vi "MPU_Stick_Plotter_Core_Test.vi"() -> ()   [LabVIEW 2017]
uses:
  <vilib>/Utility/miscctls.llb/LVPointDoubleTypeDef.ctl
  <vilib>/Utility/miscctls.llb/LVOffsetAndMultiplierTypeDef.ctl
  Controls/MPU_Stick_Plotter_Core_Commands.ctl
panel:
  out "Plot":cluster{"Values":dbl[], "Time (ms)":dbl[]}[](graph)
  in  "Channel Name":string="Channel A"
  in  "Offset & Range":T1
  out "Sample value":dbl
  out "Cursor.Cursor Position":T2
  in  "stop":bool
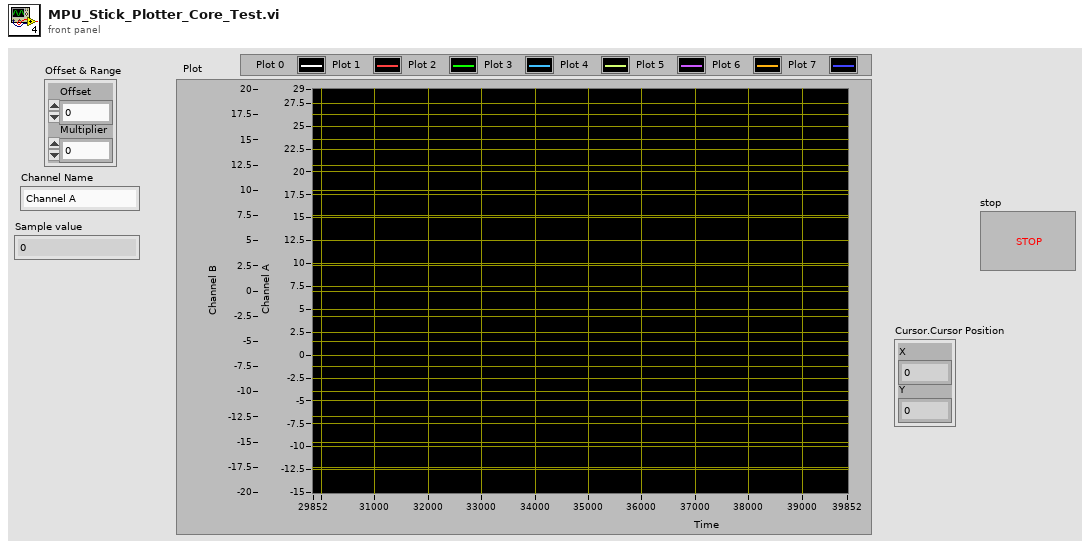
[diagram p1: front panel]
types:
  T1 = typedef "LVOffsetAndMultiplierTypeDef.ctl" = cluster{"Offset":dbl, "Multiplier":dbl}
  T2 = typedef "LVPointDoubleTypeDef.ctl" = cluster{"X":dbl, "Y":dbl}
  T3 = typedef "MPU_Stick_Plotter_Core_Commands.ctl" = enum16{"Initialize", "Add Channel", "Remove Channel", "Set Channel Minimum Value", "Set Channel Maximum Value", "Set Offset & Multiplier", "Get Offset & Multiplier", "Update Channel", "Get Cursor Data", "Clear", "Reset"}
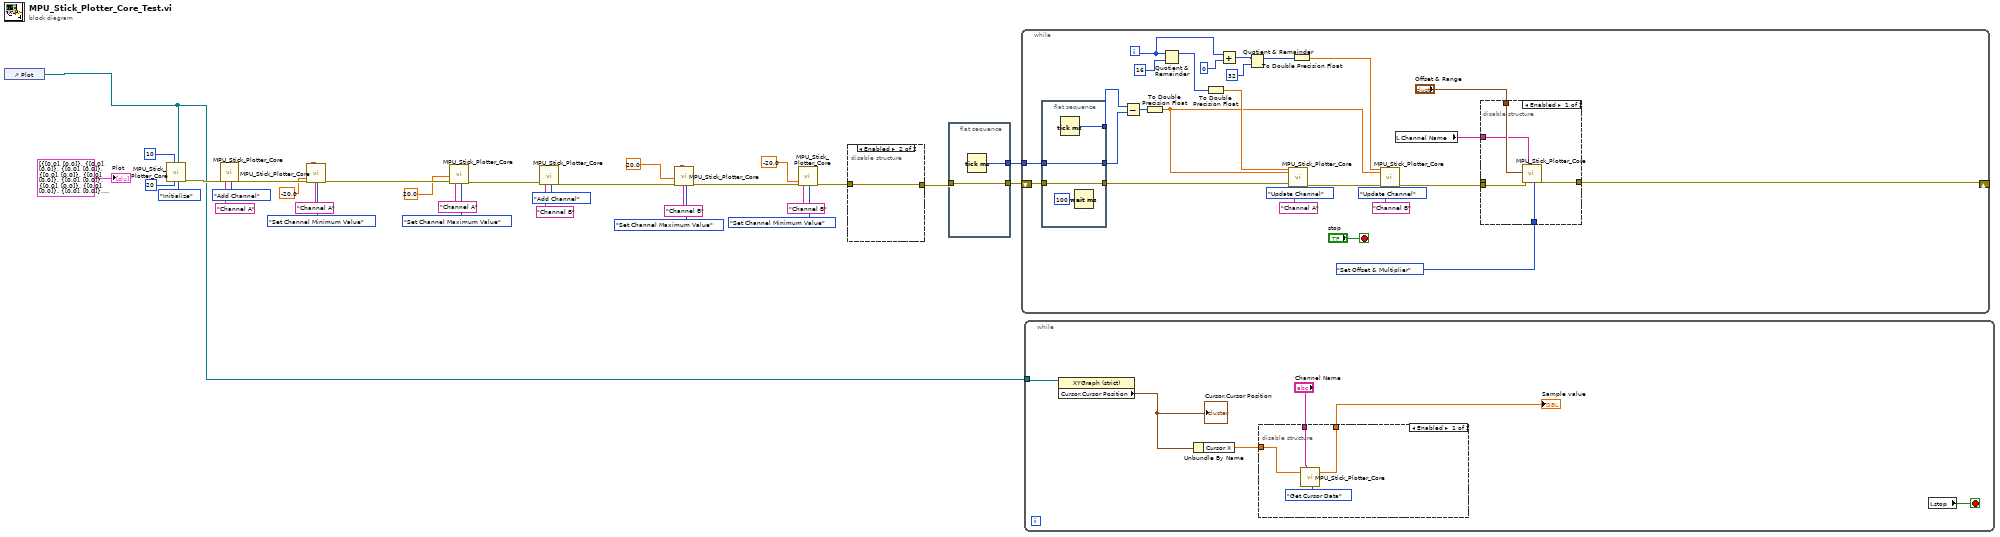
[diagram p0: block diagram]
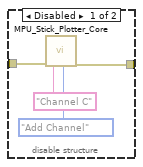
[diagram p2: hidden frame]
diagram:
  n1 = control-ref of="Plot"() -> (w1:refnum<vi>)
  n2 = call "MPU_Stick_Plotter_Core.vi"("Number of vertical divisions"=u16 10, "Number of horizontal divisions"=u16 20, "Plot reference"=w1, "Command"=MPU_Stick_Plotter_Core_Commands."Initialize") -> ("error out"=w30:errorcluster)  [unwired: 12 in, 3 out]
  n3 = call "MPU_Stick_Plotter_Core.vi"("error in (no error)"=w30, "Channel Name"="Channel A", "Command"=MPU_Stick_Plotter_Core_Commands."Add Channel") -> ("error out"=w25:errorcluster)  [unwired: 13 in, 3 out]
  n4 = call "MPU_Stick_Plotter_Core.vi"("Minimum"=-20.0, "error in (no error)"=w25, "Channel Name"="Channel A", "Command"=MPU_Stick_Plotter_Core_Commands."Set Channel Minimum Value") -> ("error out"=w21:errorcluster)  [unwired: 12 in, 3 out]
  n5 = call "MPU_Stick_Plotter_Core.vi"("Maximum"=20.0, "error in (no error)"=w21, "Channel Name"="Channel A", "Command"=MPU_Stick_Plotter_Core_Commands."Set Channel Maximum Value") -> ("error out"=w11:errorcluster)  [unwired: 12 in, 3 out]
  n6 = call "MPU_Stick_Plotter_Core.vi"("error in (no error)"=w11, "Channel Name"="Channel B", "Command"=MPU_Stick_Plotter_Core_Commands."Add Channel") -> ("error out"=w17:errorcluster)  [unwired: 13 in, 3 out]
  n7 = call "MPU_Stick_Plotter_Core.vi"("Maximum"=20.0 ("Units / division"), "error in (no error)"=w17, "Channel Name"="Channel B", "Command"=MPU_Stick_Plotter_Core_Commands."Set Channel Maximum Value") -> ("error out"=w14:errorcluster)  [unwired: 12 in, 3 out]
  n8 = call "MPU_Stick_Plotter_Core.vi"("Minimum"=-20.0 ("Offset (units)"), "error in (no error)"=w14, "Channel Name"="Channel B", "Command"=MPU_Stick_Plotter_Core_Commands."Set Channel Minimum Value") -> ("error out"=w4:errorcluster)  [unwired: 12 in, 3 out]
  n9 = disable-structure shown="Enabled" {
    disable-tunnel: w4 -> [w35 w36]
    disable-tunnel: [w34 w36] -> w3
    frame Disabled {
      n10 = call "MPU_Stick_Plotter_Core.vi"("error in (no error)"=w35, "Channel Name"="Channel C", "Command"=MPU_Stick_Plotter_Core_Commands."Add Channel") -> ("error out"=w34:errorcluster)  [unwired: 13 in, 3 out]
    }
    frame Enabled {
    }
  }
  n11 = flat-sequence {
    tunnel: w3 -> [w38]
    tunnel: [w38] -> w27
    tunnel: [w37] -> w26
    frame #0 {
      n12 = Tick Count (ms)() -> (millisecond timer value=w37:u32)
    }
  }
  n13 = while {
    tunnel: w26 -> [w59]
    shift-right: [w41] -> _
    shift-left: w27 -> [w64]
    i -> [w44]
    stop <- "stop" stop-if-true
    n14 = flat-sequence {
      tunnel: w64 -> [w75]
      tunnel: [w75] -> w63
      tunnel: [w73] -> w60
      tunnel: w59 -> [w72]
      tunnel: [w72] -> w58
      frame #0 {
        n15 = Tick Count (ms)() -> (millisecond timer value=w73:u32)
        n16 = Wait (ms)(milliseconds to wait=u32 100) -> ()  [unwired: 1 out]
      }
    }
    n17 = Subtract(x=w60, y=w58) -> (x-y=w57:u32)
    n18 = To Double Precision Float(number=w57) -> (double precision float=w49:dbl)
    n19 = Quotient & Remainder(x=w44, y=16) -> (x-y*floor(x/y)=w54:i32)  [unwired: 1 out]
    n20 = To Double Precision Float(number=w54) -> (double precision float=w55:dbl)
    n21 = Add(x=w44, y=0) -> (x+y=w47:i32)
    n22 = Quotient & Remainder(x=w47, y=32) -> (x-y*floor(x/y)=w45:i32)  [unwired: 1 out]
    n23 = call "MPU_Stick_Plotter_Core.vi"("Value (original)"=w55, "Time (ms)"=w49, "error in (no error)"=w63, "Channel Name"="Channel A", "Command"=MPU_Stick_Plotter_Core_Commands."Update Channel") -> ("error out"=w50:errorcluster)  [unwired: 11 in, 3 out]
    n24 = To Double Precision Float(number=w45) -> (double precision float=w48:dbl)
    n25 = call "MPU_Stick_Plotter_Core.vi"("Value (original)"=w48, "Time (ms)"=w49, "error in (no error)"=w50, "Channel Name"="Channel B", "Command"=MPU_Stick_Plotter_Core_Commands."Update Channel") -> ("error out"=w40:errorcluster)  [unwired: 11 in, 3 out]
    n26 = local read "Channel Name"() -> (w39:string)
    n27 = disable-structure shown="Enabled" {
      disable-tunnel: _ -> [_ w71]
      disable-tunnel: MPU_Stick_Plotter_Core_Commands."Set Offset & Multiplier" ("Command") -> [w70 _]
      disable-tunnel: "Offset & Range" -> [w69 _]
      disable-tunnel: [w68 w71] -> w41
      disable-tunnel: w40 -> [w67 _]
      disable-tunnel: w39 -> [w66 _]
      frame Enabled {
        n28 = call "MPU_Stick_Plotter_Core.vi"("Offset & Multiplier"=w69, "error in (no error)"=w67, "Channel Name"=w66, "Command"=w70) -> ("error out"=w68:errorcluster)  [unwired: 12 in, 3 out]
      }
      frame Disabled {
      }
    }
  }
  n29 = while {
    tunnel: w1 -> [w80]
    stop <- w81 stop-if-true
    n30 = property class="XYGraph (strict)"(reference=w80) -> ("Cursor.Cursor Position"=w79:T2)  [unwired: 1 in, 2 out]
    "Cursor.Cursor Position" <- w79
    n31 = Unbundle By Name(w79) -> ("Cursor X"=w78:dbl)
    n32 = disable-structure shown="Enabled" {
      disable-tunnel: w78 -> [w84 _]
      disable-tunnel: [w83 _] -> w77
      disable-tunnel: "Channel Name" -> [w82 _]
      frame Enabled {
        n33 = call "MPU_Stick_Plotter_Core.vi"("Time (ms)"=w84, "Channel Name"=w82, "Command"=MPU_Stick_Plotter_Core_Commands."Get Cursor Data") -> ("Sample value"=w83:dbl)  [unwired: 13 in, 3 out]
      }
      frame Disabled {
      }
    }
    "Sample value" <- w77
    n34 = local read "stop"() -> (w81:bool)
  }
  "Plot" <- cluster{"Value":dbl[], "Time (ms)":dbl[]}[] [{"Value"=[0.0], "Time (ms)"=[0.0]}, {"Value"=[0.0], "Time (ms)"=[0.0]}, {"Value"=[0.0], "Time (ms)"=[0.0]}, {"Value"=[0.0], "Time (ms)"=[0.0]}, {"Value"=[0.0], "Time (ms)"=[0.0]}, {"Value"=[0.0], "Time (ms)"=[0.0]}, {"Value"=[0.0], "Time (ms)"=[0.0]}, {"Value"=[0.0], "Time (ms)"=[0.0]}, {"Value"=[0.0], "Time (ms)"=[0.0]}, {"Value"=[0.0], "Time (ms)"=[0.0]}, {"Value"=[0.0], "Time (ms)"=[0.0]}, {"Value"=[0.0], "Time (ms)"=[0.0]}, {"Value"=[0.0], "Time (ms)"=[0.0]}, {"Value"=[0.0], "Time (ms)"=[0.0]}, {"Value"=[0.0], "Time (ms)"=[0.0]}, {"Value"=[0.0], "Time (ms)"=[0.0]}, {"Value"=[0.0], "Time (ms)"=[0.0]}, {"Value"=[0.0], "Time (ms)"=[0.0]}, {"Value"=[0.0], "Time (ms)"=[0.0]}, {"Value"=[0.0], "Time (ms)"=[0.0]}, {"Value"=[0.0], "Time (ms)"=[0.0]}, {"Value"=[0.0], "Time (ms)"=[0.0]}, {"Value"=[0.0], "Time (ms)"=[0.0]}, {"Value"=[0.0], "Time (ms)"=[0.0]}, {"Value"=[0.0], "Time (ms)"=[0.0]}, {"Value"=[0.0], "Time (ms)"=[0.0]}, {"Value"=[0.0], "Time (ms)"=[0.0]}, {"Value"=[0.0], "Time (ms)"=[0.0]}, {"Value"=[0.0], "Time (ms)"=[0.0]}, {"Value"=[0.0], "Time (ms)"=[0.0]}, {"Value"=[0.0], "Time (ms)"=[0.0]}, {"Value"=[0.0], "Time (ms)"=[0.0]}] ("XY Graph")
